vi "Evaluate Partial Derivatives of 2-Exp.vi"(8 "error in (no error)":errorcluster, 9 "Ramp":dbl[](array[numeric]), 10 "Fitted Parameter Names":T2[](array[typedef]), 11 "1-Exp Parameters Array":T3[](array[typedef])) -> (0 "error out":errorcluster, 3 "Partial Derivatives Plot Array":T1[](array[typedef]))   [LabVIEW 2021, in "Fits.lvlib"]
uses:
  Fits.lvlib
  1-Exp Parameters.ctl
  IRF(X)PSED/Decay Fit Parameters In List.ctl
  Graphs/XY Graph/XY Graph Plot Data.ctl
  a24067bf-37e1-4c88-a2d0-01b8de0df140.vi
  Graphs/XY Graph/XY Graph Add-Ons.lvlib
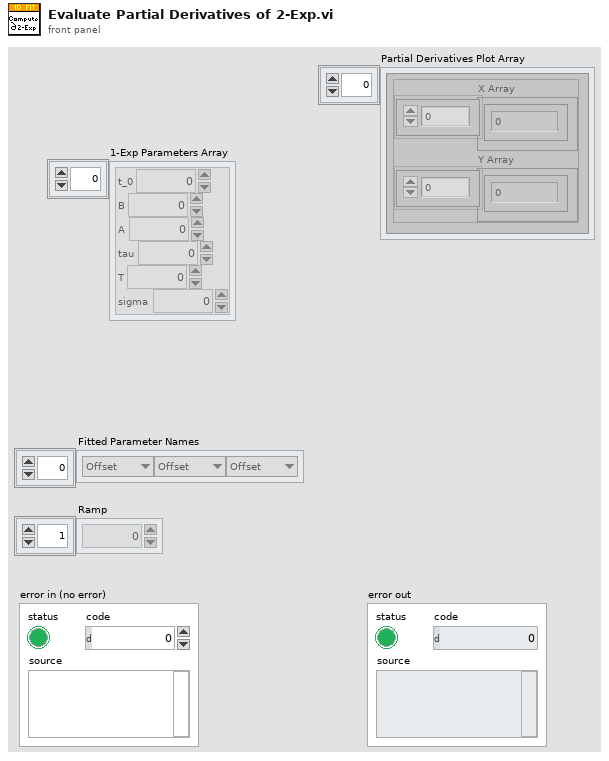
[diagram p1: front panel]
types:
  T1 = typedef "XY Graph Add-Ons.lvlib/XY Graph Plot Data.ctl" = cluster{"X Array":dbl[], "Y Array":dbl[]}
  T2 = typedef "Fits.lvlib/Decay Fit Parameters In List.ctl" = enum16{"Offset", "Baseline", "A_1", "tau_1", "A_2", "tau_2"}
  T3 = typedef "Fits.lvlib/1-Exp Parameters.ctl" = cluster{"t_0":dbl, "B":dbl, "A":dbl, "tau":dbl, "T":dbl, "sigma":dbl}
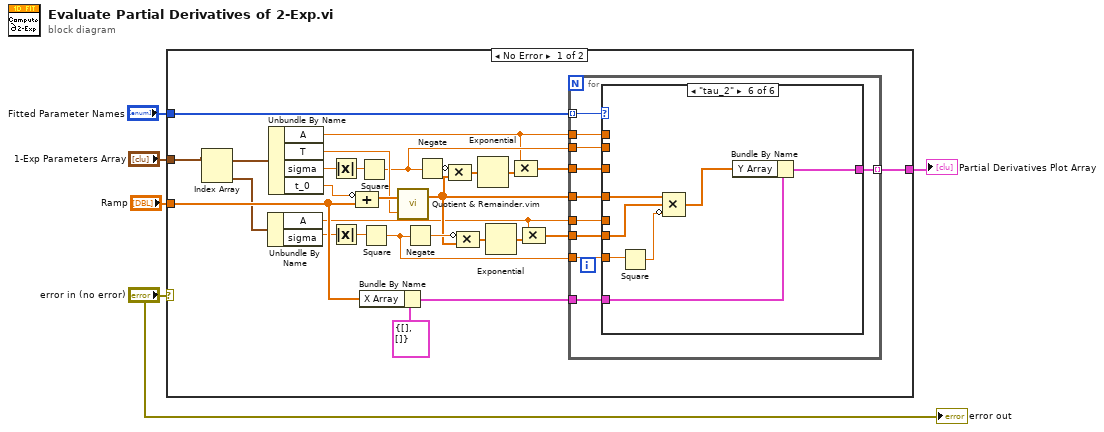
[diagram p0: block diagram]
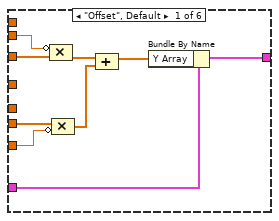
[diagram p2: hidden frame]
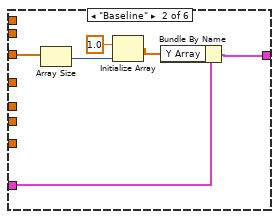
[diagram p3: hidden frame]
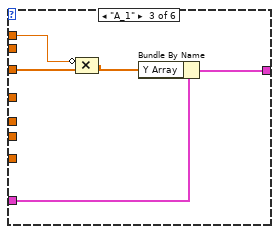
[diagram p4: hidden frame]
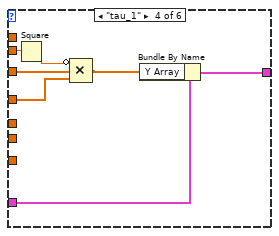
[diagram p5: hidden frame]
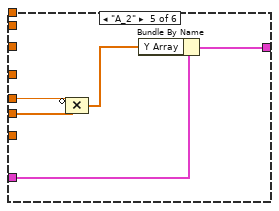
[diagram p6: hidden frame]
diagram:
  n1 = case shown="No Error" "error in (no error)" {
    tunnel: "1-Exp Parameters Array" -> [w19 _]
    tunnel: "Ramp" -> [w26 _]
    tunnel: "Fitted Parameter Names" -> [w27 _]
    tunnel: [w21 _] -> w1
    frame No Error {
      n2 = Index Array(array=w19) -> (element #1=w20:T3, element #2=w18:T3)  [unwired: 2 in]
      n3 = Unbundle By Name(w18) -> ("A"=w12:dbl, "sigma"=w11:dbl)
      n4 = Unbundle By Name(w20) -> ("A"=w6:dbl, "T"=w31:dbl, "sigma"=w22:dbl, "t_0"=w33:dbl)
      n5 = Absolute Value(x=w22) -> (abs(x)=w10:dbl)
      n6 = Absolute Value(x=w11) -> (abs(x)=w8:dbl)
      n7 = Compound Arithmetic op=ADD(invert w33, w26) -> (w32:dbl[])
      n8 = Square(x=w10) -> (x^2=w9:dbl)
      n9 = Bundle By Name(cluster=T1 {"X Array"=[], "Y Array"=[]} ("Plot"), "X Array"=w26) -> (w24:T1)
      n10 = Square(x=w8) -> (x^2=w7:dbl)
      n11 = call "Quotient & Remainder.vim"("y"=w31, "x"=w32) -> ("x - E(x/y)y"=w14:dbl[])  [unwired: 1 out]
      n12 = Negate(x=w7) -> (-x=w17:dbl)
      n13 = Negate(x=w9) -> (-x=w28:dbl)
      n14 = Compound Arithmetic op=MULTIPLY(invert w28, w14) -> (w30:dbl[])
      n15 = Compound Arithmetic op=MULTIPLY(invert w17, w14) -> (w15:dbl[])
      n16 = Exponential(1:w30) -> (0:w29:dbl[])
      n17 = Exponential(1:w15) -> (0:w16:dbl[])
      n18 = Compound Arithmetic op=MULTIPLY(w6, w29) -> (w23:dbl[])
      n19 = Compound Arithmetic op=MULTIPLY(w12, w16) -> (w13:dbl[])
      n20 = for {
        tunnel: w27 -> [w43] mode=indexing
        tunnel: w24 -> [w42]
        tunnel: w23 -> [w41]
        tunnel: w9 -> [w40]
        tunnel: w14 -> [w39]
        tunnel: [w38] -> w21 mode=indexing
        tunnel: w13 -> [w37]
        tunnel: w12 -> [w36]
        tunnel: w7 -> [w35]
        tunnel: w6 -> [w34]
        n21 = case shown="\"tau_2\"" w43 {
          tunnel: w42 -> [w49 w53 w61 w66 w74 w81]
          tunnel: w41 -> [w52 w58 w63 w70 _ _]
          tunnel: w40 -> [w51 _ _ w69 _ _]
          tunnel: [w48 w54 w60 w64 w73 w79] -> w38
          tunnel: w39 -> [_ _ _ w67 _ w82]
          tunnel: w37 -> [w47 _ _ _ w72 w78]
          tunnel: w36 -> [_ _ _ _ w71 _]
          tunnel: w35 -> [w46 _ _ _ _ w77]
          tunnel: w34 -> [_ _ w59 _ _ _]
          frame "Offset", Default {
            n22 = Compound Arithmetic op=MULTIPLY(invert w51, w52) -> (w50:dbl[])
            n23 = Compound Arithmetic op=MULTIPLY(w47, invert w46) -> (w44:dbl[])
            n24 = Compound Arithmetic op=ADD(w50, w44) -> (w45:dbl[])
            n25 = Bundle By Name(cluster=w49, "Y Array"=w45) -> (w48:T1)
          }
          frame "Baseline" {
            n26 = Array Size(array=w58) -> (size(s)=w57:i32)
            n27 = Initialize Array(1.0 ("element"), w57) -> (w55:dbl[])
            n28 = Bundle By Name(cluster=w53, "Y Array"=w55) -> (w54:T1)
          }
          frame "A_1" {
            n29 = Compound Arithmetic op=MULTIPLY(invert w59, w63) -> (w62:dbl[])
            n30 = Bundle By Name(cluster=w61, "Y Array"=w62) -> (w60:T1)
          }
          frame "tau_1" {
            n31 = Square(x=w69) -> (x^2=w68:dbl)
            n32 = Compound Arithmetic op=MULTIPLY(invert w68, w70, w67) -> (w65:dbl[])
            n33 = Bundle By Name(cluster=w66, "Y Array"=w65) -> (w64:T1)
          }
          frame "A_2" {
            n34 = Compound Arithmetic op=MULTIPLY(invert w71, w72) -> (w75:dbl[])
            n35 = Bundle By Name(cluster=w74, "Y Array"=w75) -> (w73:T1)
          }
          frame "tau_2" {
            n36 = Square(x=w77) -> (x^2=w76:dbl)
            n37 = Compound Arithmetic op=MULTIPLY(w82, w78, invert w76) -> (w80:dbl[])
            n38 = Bundle By Name(cluster=w81, "Y Array"=w80) -> (w79:T1)
          }
        }
      }
    }
    frame Error {
    }
  }
  "Partial Derivatives Plot Array" <- w1
  "error out" <- "error in (no error)"
